vi "DEMO.vi"() -> ()   [LabVIEW 2013, in "Management Ojbect Searcher.lvlib"]
uses:
  Management Ojbect Searcher.lvlib
  Query String.ctl
panel:
  in  "QueryString":T1
  out "Info":string[](array[string])
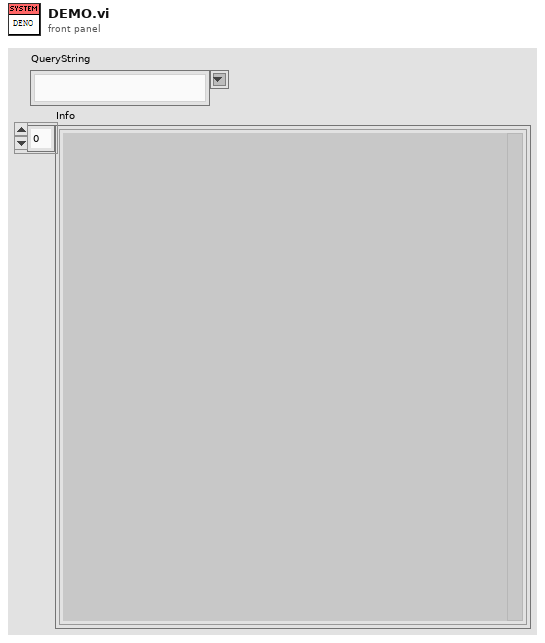
[diagram p1: front panel]
types:
  T1 = typedef "Management Ojbect Searcher.lvlib/Query String.ctl" = string
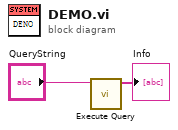
[diagram p0: block diagram]
diagram:
  n1 = call "Execute Query.vi"("QueryString"="QueryString") -> ("Info"=→"Info":string[])  [unwired: 9 in, 1 out]
